vi "AlliGator Get I-m-phi Dataset Phasor Harmonic Components.vi"(8 "Error In":errorcluster, 11 "Harmonic Data":T1[](array[typedef])) -> (0 "Error Out":errorcluster, 1 "Harmonic Order":u8[](array[numeric]), 3 "Phasor Components":sgl[][][](array[numeric]))   [LabVIEW 2021, in "AlliGator Files.lvlib"]
doc: "Converts FLIMBox data structure to one used internally in AlliGator."
uses:
  AlliGator Files.lvlib
  FLIMbox/FLIMbox Harmonic Data.ctl
  FLIMbox/FLIMBox.lvlib
panel:
  # "see the AlliGator License on the block diagram (Ctrl+E or Window:Show Block Diagram)"
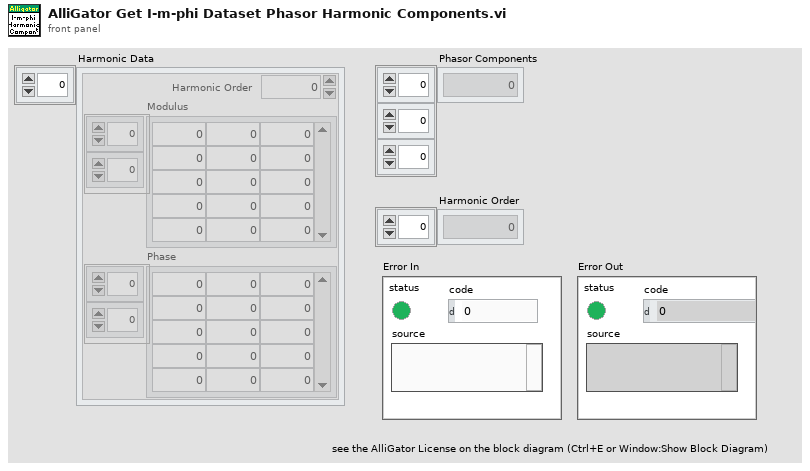
[diagram p1: front panel]
types:
  T1 = typedef "FLIMBox.lvlib/FLIMbox Harmonic Data.ctl" = cluster{"Modulus":sgl[][], "Phase":sgl[][], "Harmonic Order":u8}
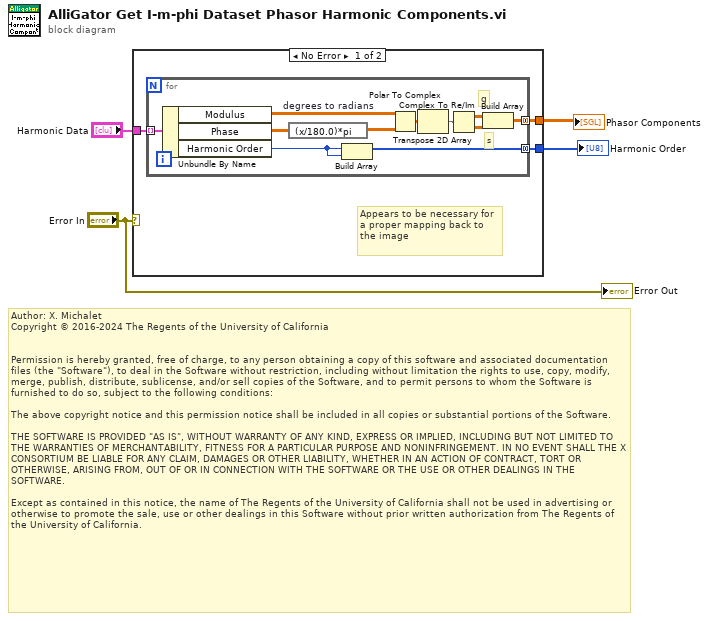
[diagram p0: block diagram]
diagram:
  # "Author: X. Michalet\nCopyright © 2016-2024 The Regents of the University of California\n \n\nPermission is hereby granted, free of charge, to any person obtaining a copy of this software and associated documentation files (the \"Software\"), to deal in the Software without restriction, including without limitation the rights to use, copy, modify, merge, publish, distribute, sublicense, and/or sell copies of the Software, and to permit persons to whom the Software is furnished to do so, subject to the following conditions:\n\nThe above copyright notice and this permission notice shall be included in all copies or substantial portions of the Software.\n\nTHE SOFTWARE IS PROVIDED \"AS IS\", WITHOUT WARRANTY OF ANY KIND, EXPRESS OR IMPLIED, INCLUDING BUT NOT LIMITED TO THE WARRANTIES OF MERCHANTABILITY, FITNESS FOR A PARTICULAR PURPOSE AND NONINFRINGEMENT. IN NO EVENT SHALL THE X CONSORTIUM BE LIABLE FOR ANY CLAIM, DAMAGES OR OTHER LIABILITY, WHETHER IN AN ACTION OF CONTRACT, TORT OR OTHERWISE, ARISING FROM, OUT OF OR IN CONNECTION WITH THE SOFTWARE OR THE USE OR OTHER DEALINGS IN THE SOFTWARE.\n\nExcept as contained in this notice, the name of The Regents of the University of California shall not be used in advertising or otherwise to promote the sale, use or other dealings in this Software without prior written authorization from The Regents of the University of California."
  n1 = case shown="No Error" "Error In" {
    tunnel: "Harmonic Data" -> [w7 _]
    tunnel: [w6 _] -> w3
    tunnel: [w5 _] -> w1
    frame No Error {
      # "Appears to be necessary for a proper mapping back to  the image"
      n2 = for {
        tunnel: w7 -> [w18] mode=indexing
        tunnel: [w16] -> w6 mode=concatenating
        tunnel: [w10] -> w5 mode=concatenating
        # "s"
        # "g"
        n3 = Unbundle By Name(w18) -> ("Modulus"=w13:sgl[][], "Phase"=w15:sgl[][], "Harmonic Order"=w17:u8)
        n4 = expression code="(x/180.0)*pi" "degrees to radians"(w15) -> (w14:sgl[][])
        n5 = Build Array(w17, w17) -> (w16:u8[])
        n6 = Polar To Complex(1:w14, 2:w13) -> (0:w12:csg[][])
        n7 = Transpose 2D Array(2D array=w12) -> (transposed array=w8:csg[][])
        n8 = Complex To Re/Im(x + iy=w8) -> (x=w11:sgl[][], y=w9:sgl[][])
        n9 = Build Array(w11, w9) -> (w10:sgl[][][])
      }
    }
    frame Error {
    }
  }
  "Harmonic Order" <- w3
  "Phasor Components" <- w1
  "Error Out" <- "Error In"
